vi "Write RH.vi"(8 "error in (no error)":errorcluster, 10 "RH":dbl, 11 "humData in":refnum<class "humData.lvclass">) -> (0 "error out":errorcluster, 3 "humData out":refnum<class "humData.lvclass">)   [LabVIEW 2014, in "humData.lvclass"]
uses:
  humData.lvclass
  humData.lvclass/humData.ctl
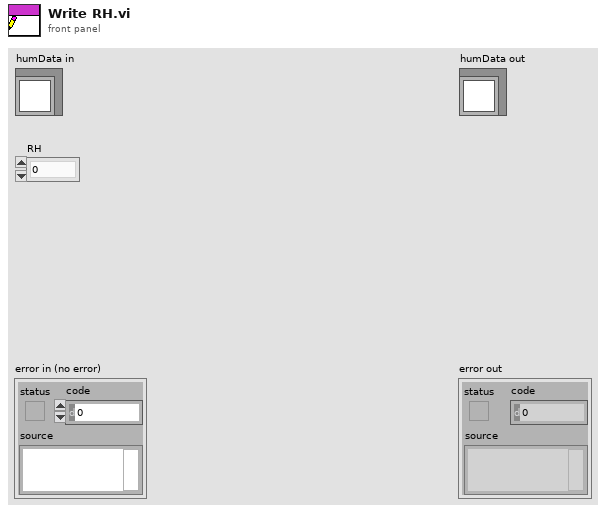
[diagram p1: front panel]
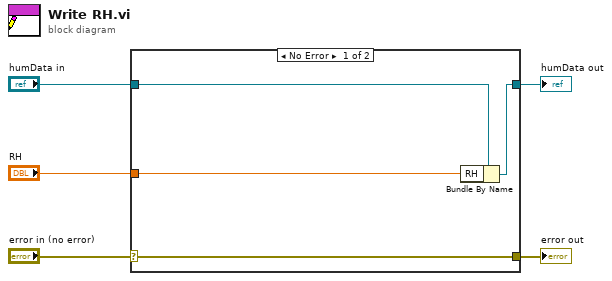
[diagram p0: block diagram]
diagram:
  n1 = case shown="No Error" "error in (no error)" {
    selector: "error in (no error)" -> [w9 w10]
    tunnel: [w9 w10] -> w4
    tunnel: [w7 w11] -> w2
    tunnel: "humData in" -> [w8 w11]
    tunnel: "RH" -> [w6 _]
    frame No Error {
      n2 = Bundle By Name(cluster=w8, "RH"=w6) -> (w7:refnum<class "humData.lvclass">)
    }
    frame Error {
    }
  }
  "error out" <- w4
  "humData out" <- w2
